vi "Set User Event.vi"(11 "userEvent":u32) -> (2 "function return":u32, 3 "userEvent out":u32)   [LabVIEW 2018, in "Copy of Andor SDK.lvlib"]
doc: "EXPNETTYPE unsigned int WINAPI SetUserEvent(HANDLE userEvent);"
uses:
  Copy of Andor SDK.lvlib
  <userlib>/Andor SDK/ATMCD32D.dll
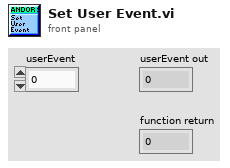
[diagram p1: front panel]
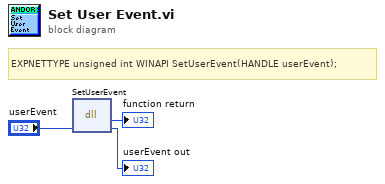
[diagram p0: block diagram]
diagram:
  # "EXPNETTYPE unsigned int WINAPI SetUserEvent(HANDLE userEvent);"
  n1 = dll-call lib="C:/Program Files (x86)/National Instruments/LabVIEW 2018/user.lib/Andor SDK/ATMCD32D.*" fn="SetUserEvent"("userEvent"="userEvent") -> (→"function return":u32, "userEvent"=→"userEvent out":u32)  [unwired: 3 in, 2 out]
